vi "CAN-sender-MPS.vi"() -> ()   [LabVIEW 2011]
uses:
  <vilib>/nican/nican.llb/ncNetAttr.ctl
panel:
  in  "Set RTR flag?":bool
  in  "Send?":bool
  in  "Mode":bool
  in  "# Bytes (1 or 2)":i16=2
  in  "Data":i16
  in  "ID (0->11)":u32
  in  "Interface (usually CAN0)":string(combo)="CAN0"
  in  "stop":bool
  in  "Baudrate (usually 50000)":u32=500000
  # "HOW TO USE:\n\n1. Plug the NI USB-8473(s) modules into the CAN bus.\n2. Unplug the C8051 from the CAN bus. (This VI will be used to send commands instead of the C8051.)\n3. Hit Ctrl+R to start."
  # "STOP sending frames"
  # "Single"
  # "Continuous"
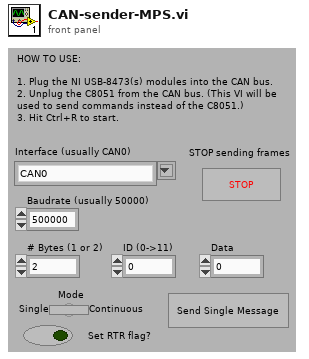
[diagram p1: front panel]
types:
  T1 = typedef "ncNetAttr.ctl" = cluster{"Start On Open":enum32{"FALSE", "TRUE"}, "Baud Rate":u32, "Read Queue Length":u32, "Write Queue Length":u32, "Standard Comparator":u32, "Standard Mask":u32, "Extended Comparator":u32, "Extended Mask":u32}
  T2 = typedef "xobjhandle.ctl" = u32
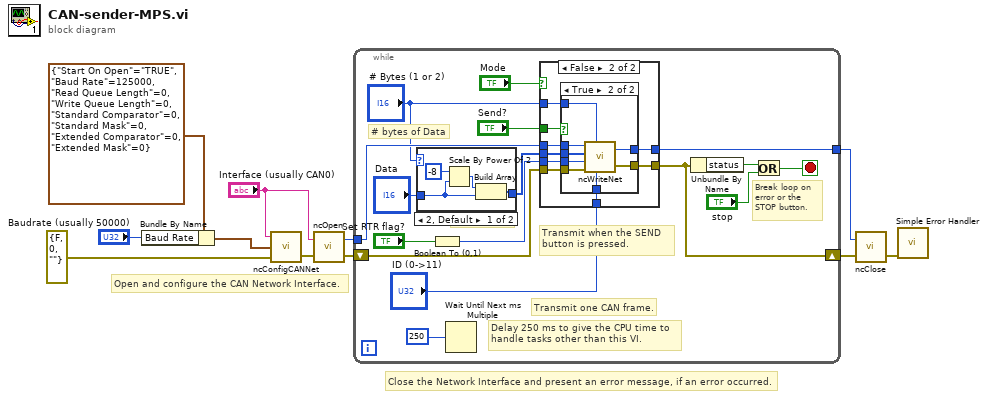
[diagram p0: block diagram]
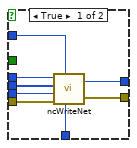
[diagram p2: hidden frame]
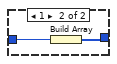
[diagram p4: hidden frame]
diagram:
  # "Open and configure the CAN Network Interface."
  # "Close the Network Interface and present an error message, if an error occurred."
  n1 = Bundle By Name(cluster=T1 {"Start On Open"=enum."TRUE", "Baud Rate"=125000, "Read Queue Length"=0, "Write Queue Length"=0, "Standard Comparator"=0, "Standard Mask"=0, "Extended Comparator"=0, "Extended Mask"=0} ("CAN Network Interface Config"), "Baud Rate"="Baudrate (usually 50000)") -> (w8:T1)
  n2 = call <vilib>:"ncConfigCANNet.vi"("Error in"=errorcluster {"status"=FALSE, "code"=0, "source"=""}, "CAN Network Interface Config"=w8, "ObjName"="Interface (usually CAN0)") -> ("Error out"=w10:errorcluster)  [unwired: 2 out]
  n3 = call <vilib>:"ncOpen.vi"("Error in"=w10, "ObjName"="Interface (usually CAN0)") -> ("Error out"=w4:errorcluster, "ObjHandle out"=w6:T2)
  n4 = while {
    shift-left: w4 -> [w14]
    shift-right: [w23] -> w3
    tunnel: w6 -> [w20]
    tunnel: [w27] -> w5
    stop <- w26 stop-if-true
    # "int->2 bytes"
    # "# bytes of Data"
    # "Transmit one CAN frame."
    # "Transmit when the SEND button is pressed."
    # "Delay 250 ms to give the CPU time to handle tasks other than this VI."
    # "Break loop on error or the STOP button."
    n5 = case shown="2, Default" "# Bytes (1 or 2)" {
      tunnel: [w57 w59] -> w19
      tunnel: "Data" -> [w56 w60]
      frame 2, Default {
        n6 = Scale By Power Of 2(n=-8, x=w56) -> (x*2^n=w55:i16)
        n7 = Build Array(w55, w56) -> (w57:i16[])
      }
      frame 1 {
        n8 = Build Array(w60) -> (w59:i16[])
      }
    }
    n9 = Boolean To (0,1)(Boolean="Set RTR flag?") -> (0, 1=w13:i16)
    n10 = Wait Until Next ms Multiple(millisecond multiple=u32 250) -> ()  [unwired: 1 out]
    n11 = case shown="False" "Mode" {
      tunnel: [w35 w44] -> w27
      tunnel: w14 -> [w34 w43]
      tunnel: [w33 w42] -> w23
      tunnel: "ID (0->11)" -> [w32 w41]
      tunnel: w13 -> [w31 w40]
      tunnel: w20 -> [w30 w39]
      tunnel: w19 -> [w29 w38]
      tunnel: "# Bytes (1 or 2)" -> [w28 w37]
      tunnel: "Send?" -> [_ w36]
      frame True {
        n12 = call <vilib>:"ncWriteNet.vi"("ArbitrationId"=w32, "DataLength"=w28, "Error in"=w34, "IsRemote"=w31, "Data"=w29, "ObjHandle in"=w30) -> ("Error out"=w33:errorcluster, "ObjHandle out"=w35:T2)
      }
      frame False {
        n13 = case shown="True" w36 {
          tunnel: [w46 w54] -> w44
          tunnel: w43 -> [w45 w53]
          tunnel: [w45 w52] -> w42
          tunnel: w41 -> [_ w51]
          tunnel: w40 -> [_ w50]
          tunnel: w39 -> [w46 w49]
          tunnel: w38 -> [_ w48]
          tunnel: w37 -> [_ w47]
          frame False {
          }
          frame True {
            n14 = call <vilib>:"ncWriteNet.vi"("ArbitrationId"=w51, "DataLength"=w47, "Error in"=w53, "IsRemote"=w50, "Data"=w48, "ObjHandle in"=w49) -> ("Error out"=w52:errorcluster, "ObjHandle out"=w54:T2)
          }
        }
      }
    }
    n15 = Unbundle By Name(w23) -> ("status"=w24:bool)
    n16 = Or(x=w24, y="stop") -> (x .or. y?=w26:bool)
  }
  n17 = call <vilib>:"ncClose.vi"("Error in"=w3, "ObjHandle in"=w5) -> ("Error out"=w11:errorcluster)  [unwired: 1 out]
  n18 = call <vilib>:"Simple Error Handler.vi"("error in (no error)"=w11) -> ()  [unwired: 1 in, 8 out]
